vi "Main_003.vi"() -> ()   [LabVIEW 2025]
uses:
  Utility/Universal Utility/TypeDefs_Utility/Cluster_Row-Column.ctl
  9e3f57c0-2ef8-4495-8287-c6a42a5fb955.vi
  Utility/Universal Utility/TypeDefs_Utility/ENUM_4 Directions U-D-L-R.ctl
  Utility/Universal Utility/TypeDefs_Utility/ENUM_8 Directions U-D-L-R.ctl
panel:
  out "MATCH":bool
  in  "Select Data":enum32{"Example", "Puzzle"}(tab)
  in  "EX Target":u64=29
  in  "Prime Example":u64=13195
  in  "Puzzle Prime":u64=600851475143
  in  "Puzzle Target":u64=6857
  out "Answer":u64
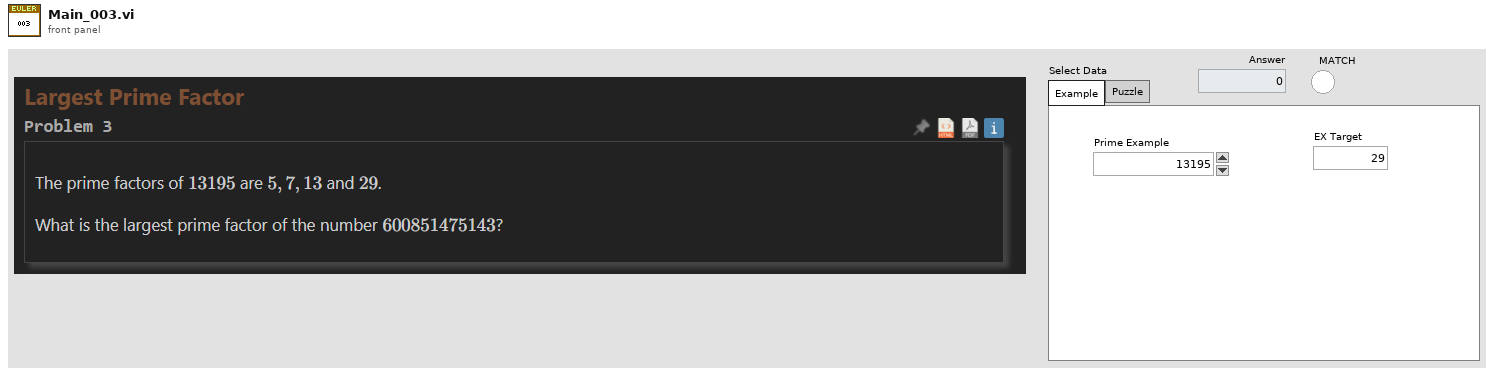
[diagram p1: front panel]
types:
  T1 = typedef "ENUM_8 Directions U-D-L-R.ctl" = enum16{"Up;-1,0", "Up-Right;-1,1", "Right;0,1", "Down-Right;1,1", "Down;1,0", "Down-Left;1,-1", "Left;0,-1", "Up-Left;-1,-1"}
  T2 = typedef "ENUM_4 Directions U-D-L-R.ctl" = enum16{"Up;-1,0", "Right;0,1", "Down;1,0", "Left;0,-1"}
  T3 = typedef "Cluster_Row-Column.ctl" = cluster{"R":i32, "C":i32}
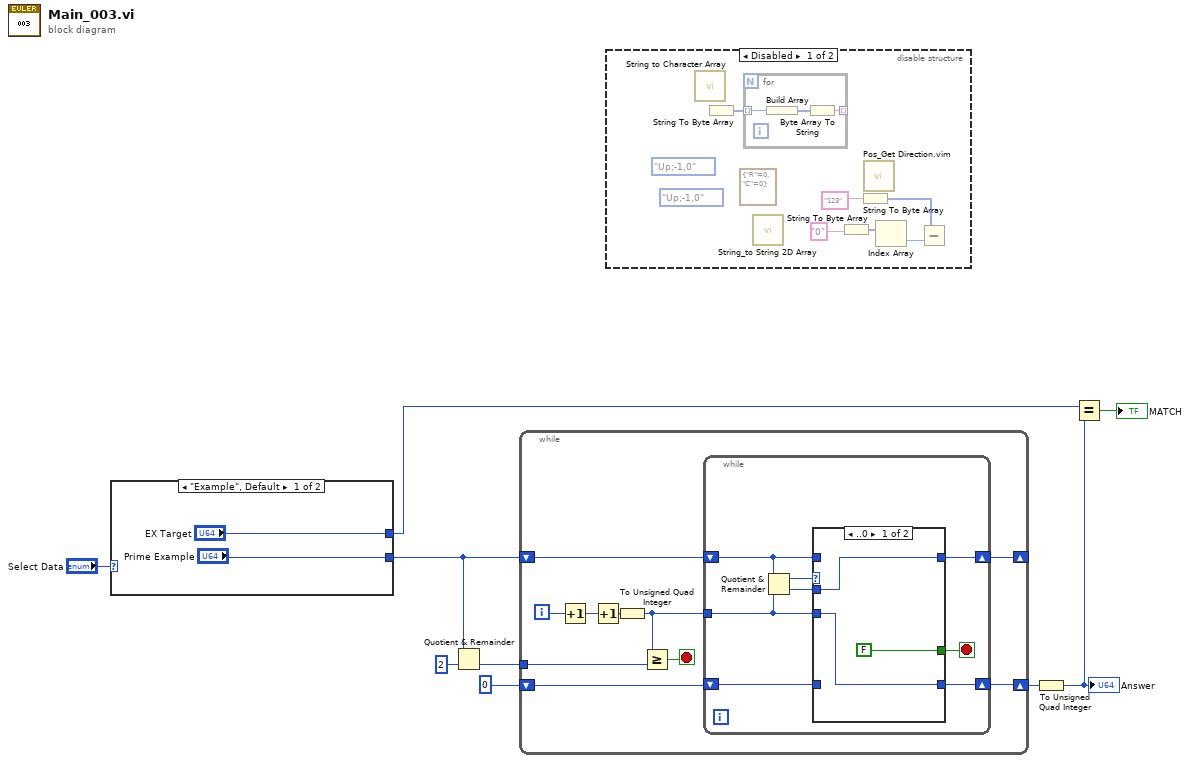
[diagram p0: block diagram]
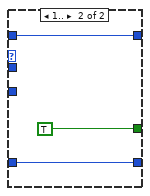
[diagram p2: hidden frame]
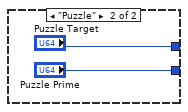
[diagram p3: hidden frame]
diagram:
  n1 = case shown="\"Example\", Default" "Select Data" {
    tunnel: ["Prime Example" "Puzzle Prime"] -> w5
    tunnel: ["EX Target" "Puzzle Target"] -> w7
    frame "Example", Default {
    }
    frame "Puzzle" {
    }
  }
  n2 = Quotient & Remainder(x=w5, y=u64 2) -> (floor(x/y)=w3:u64)  [unwired: 1 out]
  n3 = while {
    shift-right: [w20] -> _
    shift-left: w5 -> [w21]
    tunnel: w3 -> [w18]
    shift-right: [w14] -> w1
    shift-left: u64 0 ("floor(x/y)") -> [w15]
    i -> [w23]
    stop <- w17 stop-if-true
    n4 = Increment(x=w23) -> (x+1=w22:i32)
    n5 = Increment(x=w22) -> (x+1=w19:i32)
    n6 = To Unsigned Quad Integer(1:w19) -> (0:w16:u64)
    n7 = Greater Or Equal?(x=w16, y=w18) -> (x >= y?=w17:bool)
    n8 = while {
      tunnel: w16 -> [w26]
      shift-right: [w28] -> w20
      shift-left: w21 -> [w30]
      shift-right: [w27] -> w14
      shift-left: w15 -> [w25]
      stop <- w24 stop-if-true
      n9 = Quotient & Remainder(x=w30, y=w26) -> (x-y*floor(x/y)=w31:u64, floor(x/y)=w29:u64)
      n10 = case shown="..0" w31 {
        tunnel: w30 -> [_ w37]
        tunnel: w29 -> [w34 _]
        tunnel: [w34 w37] -> w28
        tunnel: [w33 w36] -> w27
        tunnel: w26 -> [w33 _]
        tunnel: w25 -> [_ w36]
        tunnel: [FALSE TRUE] -> w24
        frame ..0 {
        }
        frame 1.. {
        }
      }
    }
  }
  n11 = disable-structure shown="Disabled" {
    frame Disabled {
      (unwired) ENUM_8_Directions_U-D-L-R."Up;-1,0" ("Direction 8")
      (unwired) ENUM_4_Directions_U-D-L-R."Up;-1,0" ("Direction")
      (unwired) T3 {"R"=0, "C"=0} ("Position")
      n12 = call "String to Character Array.vi"() -> ()  [unwired: 1 in, 1 out]
      n13 = String To Byte Array() -> (unsigned byte array=w38:u8[])  [unwired: 1 in]
      n14 = for {
        tunnel: w38 -> [w46] mode=indexing
        tunnel: [w44] -> _ mode=indexing
        n15 = Build Array(w46) -> (w45:u8[])
        n16 = Byte Array To String(unsigned byte array=w45) -> (string=w44:string)
      }
      n17 = call "String_to String 2D Array.vi"() -> ()  [unwired: 11 in, 1 out]
      n18 = String To Byte Array(string="0") -> (unsigned byte array=w41:u8[])
      n19 = String To Byte Array(string="123") -> (unsigned byte array=w39:u8[])
      n20 = call "Pos_Get Direction.vim"() -> ()  [unwired: 11 in, 1 out]
      n21 = Index Array(array=w41) -> (element=w40:u8)  [unwired: 1 in]
      n22 = Subtract(x=w39, y=w40) -> ()  [unwired: 1 out]
    }
    frame Enabled {
    }
  }
  n23 = To Unsigned Quad Integer(1:w1) -> (0:w6:u64)
  "Answer" <- w6
  n24 = Equal?(x=w7, y=w6) -> (x = y?=→"MATCH":bool)
